vi "SIM limit signal (scalar).vi"(8 "limit type":T1, 9 "lower limit":dbl format="%.2f", 10 "upper limit":dbl format="%.2f", 11 "signal":dbl format="%.2f") -> (2 "limited?":bool, 3 "limited signal":dbl format="%.2f")   [LabVIEW 2024]
uses:
  SIM limit type.ctl
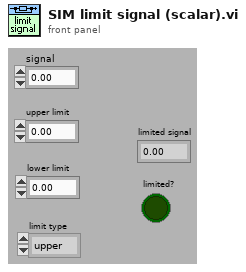
[diagram p1: front panel]
types:
  T1 = typedef "SIM limit type.ctl" = enum16{"upper", "lower", "both", "none"}
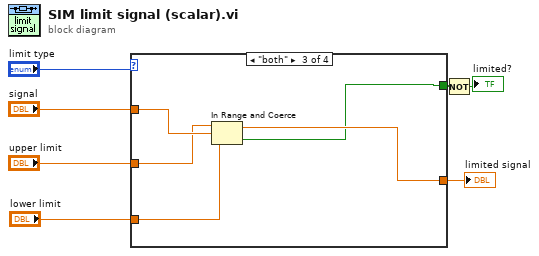
[diagram p0: block diagram]
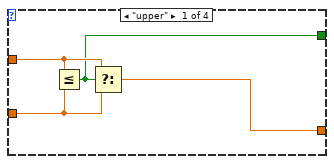
[diagram p2: hidden frame]
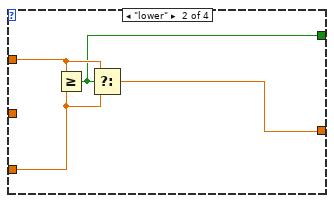
[diagram p3: hidden frame]
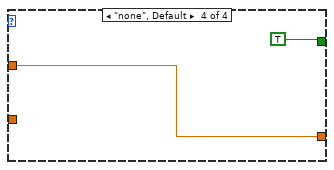
[diagram p4: hidden frame]
diagram:
  n1 = case shown="\"both\"" "limit type" {
    tunnel: "signal" -> [w11 w15 w20 w22]
    tunnel: [w9 w13 w17 w22] -> w5
    tunnel: "upper limit" -> [w10 _ w19 _]
    tunnel: "lower limit" -> [_ w14 w18 _]
    tunnel: [w8 w12 w16 TRUE] -> w2
    frame "upper" {
      n2 = Less Or Equal?(x=w11, y=w10) -> (x <= y?=w8:bool)
      n3 = Select(t=w11, s=w8, f=w10) -> (s? t:f=w9:dbl)
    }
    frame "lower" {
      n4 = Greater Or Equal?(x=w15, y=w14) -> (x >= y?=w12:bool)
      n5 = Select(t=w15, s=w12, f=w14) -> (s? t:f=w13:dbl)
    }
    frame "both" {
      n6 = In Range and Coerce(upper limit=w19, x=w20, lower limit=w18) -> (coerced(x)=w17:dbl, In Range?=w16:bool)
    }
    frame "none", Default {
    }
  }
  "limited signal" <- w5
  n7 = Not(x=w2) -> (.not. x?=→"limited?":bool)
